vi "Set Speaker Timing.vi"(8 "error in":errorcluster, 11 "cPAS in":refnum<class "cPAS.lvclass">) -> (0 "error out":errorcluster, 3 "cPAS out":refnum<class "cPAS.lvclass">)   [LabVIEW 2015, in "cPAS.lvclass"]
doc: "Check for a change in state of the speaker timing and a change in state in the speaker associated flags."
uses:
  cPAS.lvclass
  Controls/Flags.ctl
  Reusable/PAS/Main/PAS.lvclass
  Reusable/Instrument/Instrument.lvclass
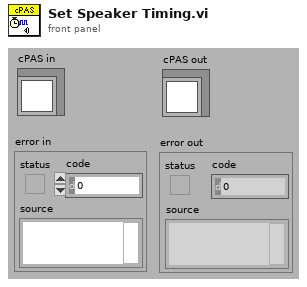
[diagram p1: front panel]
types:
  T1 = typedef "Flags.ctl" = enum8{"Autospeaker", "Link cycles", "Autofilter", "O3 Cal", "Filter Position"}
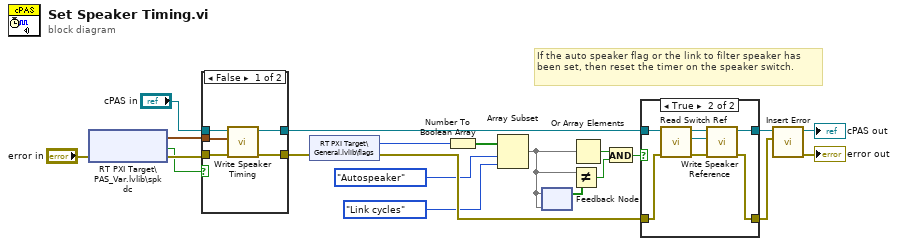
[diagram p0: block diagram]
diagram:
  # "If the auto speaker flag or the link to filter speaker has been set, then reset the timer on the speaker switch."
  n1 = shared-variable "RT PXI Target\\PAS_Var.lvlib\\spk dc"(error in="error in") -> (w17:cluster{"period":sgl, "length":sgl}, error out=w20:errorcluster, w18:bool)  [unwired: 1 in]
  n2 = case shown="False" w18 {
    tunnel: w17 -> [w22 _]
    tunnel: "cPAS in" -> [w26 w28]
    tunnel: [w25 w28] -> w13
    tunnel: w20 -> [w24 w27]
    tunnel: [w23 w27] -> w15
    frame False {
      n3 = call "Write Speaker Timing.vi"("error in"=w24, "spk dc"=w22, "PAS in"=w26) -> ("error out"=w23:errorcluster, "PAS out"=w25:refnum<class "cPAS.lvclass">)  [unwired: 7 in]
    }
    frame True {
    }
  }
  n4 = shared-variable "RT PXI Target\\General.lvlib\\flags"(error in=w15) -> (w16:u8, error out=w14:errorcluster)
  n5 = Number To Boolean Array(number=w16) -> (Boolean array=w12:bool[])
  n6 = Array Subset(array=w12, index=Flags."Autospeaker" ("Flags"), length=Flags."Link cycles" ("Flags")) -> (w8:bool[])
  n7 = feedback-in #1(w8) -> ()
  n8 = feedback #1(w8) -> (w7:bool[])
  n9 = Not Equal?(x=w8, y=w7) -> (x != y?=w10:bool)
  n10 = Or Array Elements(Boolean array=w8) -> (logical OR=w11:bool)
  n11 = And(x=w11, y=w10) -> (x .and. y?=w9:bool)
  n12 = case shown="True" w9 {
    tunnel: w14 -> [w29 w37]
    tunnel: w13 -> [w30 w33]
    tunnel: [w30 w31] -> w6
    tunnel: [w29 w32] -> w4
    frame False {
    }
    frame True {
      n13 = call "Read Switch Ref.vi"("error in"=w37, "PAS in"=w33) -> ("error out"=w35:errorcluster, "SpkSw"=w36:refnum<class "Switch.lvclass">, "PAS out"=w34:refnum<class "cPAS.lvclass">)  [unwired: 7 in]
      n14 = call "Write Speaker Reference.vi"("error in"=w35, "SpkSw"=w36, "PAS in"=w34) -> ("error out"=w32:errorcluster, "PAS out"=w31:refnum<class "cPAS.lvclass">)  [unwired: 7 in]
    }
  }
  n15 = call "Insert Error.vi"("err"=w4, "Instrument in"=w6) -> ("error out"=→"error out":errorcluster, "Instrument out"=→"cPAS out":refnum<class "cPAS.lvclass">)  [unwired: 7 in, 1 out]
